vi "Real Daq Receive.vi"(8 "error in (no error)":errorcluster, 11 "Daq Actions":T1) -> (0 "error out":errorcluster, 2 "Response Wvfms":waveform(dbl)[](array[waveform]), 3 "Responses":dbl[](array[numeric]))   [LabVIEW 2009]
uses:
  Daq Actions.ctl
  <vilib>/DAQmx/configure/timing.llb/DAQmx Timing (Sample Clock).vi
  <vilib>/DAQmx/read.llb/DAQmx Read (Analog 1D Wfm NChan 1Samp).vi
panel:
  in  "sample frequency":dbl=100.0
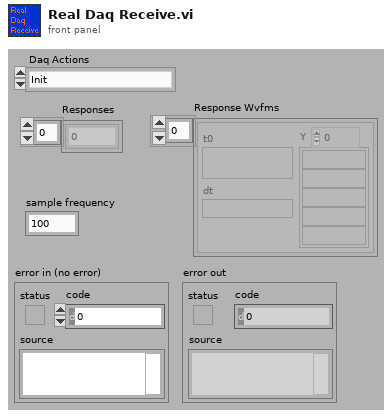
[diagram p1: front panel]
types:
  T1 = typedef "Daq Actions.ctl" = enum16{"Init", "Send Commands", "Get Responses", "Stop"}
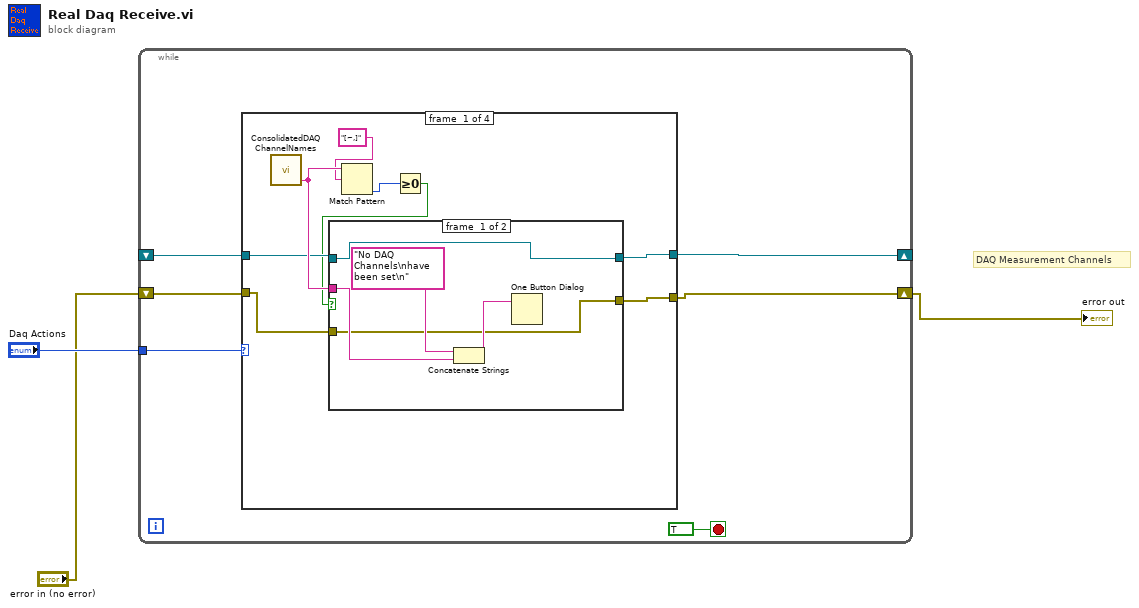
[diagram p0: block diagram]
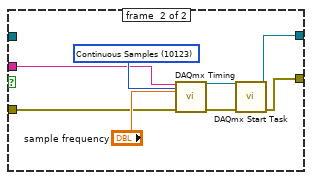
[diagram p2: hidden frame]
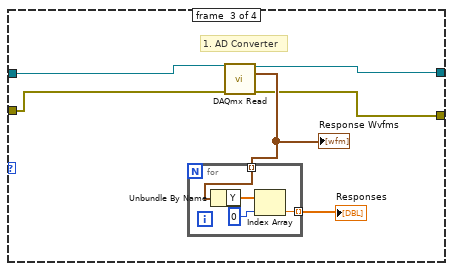
[diagram p4: hidden frame]
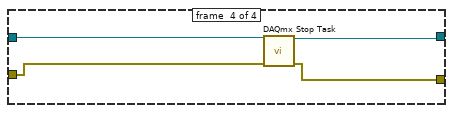
[diagram p5: hidden frame]
diagram:
  # "DAQ Measurement Channels"
  n1 = while {
    tunnel: "Daq Actions" -> [w9]
    shift-right: [w7] -> _
    shift-left: _ -> [w6]
    shift-right: [w4] -> w1
    shift-left: "error in (no error)" -> [w5]
    stop <- TRUE stop-if-true
    n2 = case shown="\"Init\"" w9 {
      tunnel: [w17 w32 w36 w45] -> w7
      tunnel: w6 -> [w12 w32 w37 w46]
      tunnel: w5 -> [w16 w31 w34 w44]
      tunnel: [w15 w31 w33 w43] -> w4
      frame #0 {
        n3 = call "ConsolidatedDAQChannelNames.vi"() -> ("Consolidated Task Names"=w14:string)  [unwired: 5 out]
        n4 = Match Pattern(string=w14, regular expression="[~,]") -> (offset past match=w13:i32)  [unwired: 4 out]
        n5 = Greater Or Equal To 0?(x=w13) -> (x >= 0?=w11:bool)
        n6 = case shown="True" w11 {
          tunnel: [w19 w27] -> w17
          tunnel: w16 -> [w18 w26]
          tunnel: [w18 w24] -> w15
          tunnel: w14 -> [w21 w23]
          tunnel: w12 -> [w19 _]
          frame #0 {
            n7 = Concatenate Strings("No DAQ Channels\nhave been set\n" ("string"), w21) -> (w22:string)
            n8 = One Button Dialog(message=w22) -> ()  [unwired: 2 out]
          }
          frame #1 {
            w29 = 10123 items=["Finite Samples"=10178, "Continuous Samples"=10123] ("sample mode")
            n9 = call-poly <vilib>:"DAQmx Timing.vi"("task/channels in"=w23, "sample mode"=w29, "rate"="sample frequency", "error in"=w26) -> ("task out"=w30:refnum<k21>, "error out"=w25:errorcluster)  [unwired: 3 in, 7 out]
            n10 = call <vilib>:"DAQmx Start Task.vi"("task/channels in"=w30, "error in"=w25) -> ("task out"=w27:refnum<k21>, "error out"=w24:errorcluster)  [unwired: 12 out]
          }
        }
      }
      frame #1 {
      }
      frame #2 {
        # "1. AD Converter"
        n11 = call-poly <vilib>:"DAQmx Read.vi"("task/channels in"=w37, "error in"=w34) -> ("task out"=w36:refnum<k21>, "data"=w38:waveform(dbl)[], "error out"=w33:errorcluster)  [unwired: 1 in, 10 out]
        "Response Wvfms" <- w38
        n12 = for {
          tunnel: w38 -> [w40] mode=indexing
          tunnel: [w39] -> w35 mode=indexing
          n13 = Unbundle By Name(w40) -> ("Y"=w41:dbl[])
          n14 = Index Array(array=w41, index=0) -> (element=w39:dbl)
        }
        "Responses" <- w35
      }
      frame #3 {
        n15 = call <vilib>:"DAQmx Stop Task.vi"("task/channels in"=w46, "error in"=w44) -> ("task out"=w45:refnum<k21>, "error out"=w43:errorcluster)  [unwired: 12 out]
      }
    }
  }
  "error out" <- w1
